vi "read_attributes.vi"(8 "error in (no error)":errorcluster, 11 "FastICA in":refnum<class "FastICA.lvclass">) -> (0 "error out":errorcluster, 2 "attributes":T1, 3 "FastICA out":refnum<class "FastICA.lvclass">)   [LabVIEW 2020, in "FastICA.lvclass"]
uses:
  FastICA.lvclass
  Controls/fast_ica_attributes.ctl
  FastICA.lvclass/FastICA.ctl
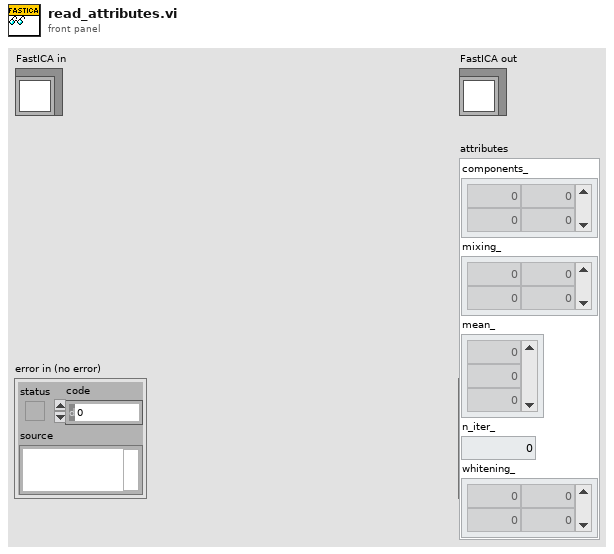
[diagram p1: front panel]
types:
  T1 = typedef "fast_ica_attributes.ctl" = cluster{"components_":dbl[][], "mixing_":dbl[][], "mean_":dbl[], "n_iter_":dbl, "whitening_":dbl[][]}
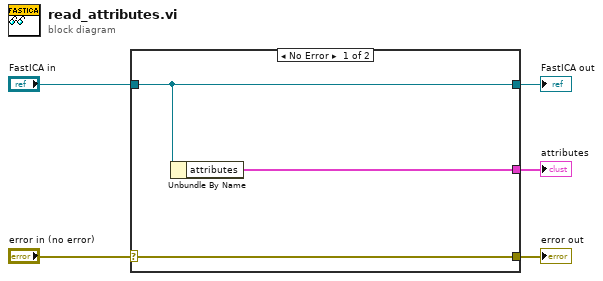
[diagram p0: block diagram]
diagram:
  n1 = case shown="No Error" "error in (no error)" {
    selector: "error in (no error)" -> [w8 w9]
    tunnel: [w8 w9] -> w4
    tunnel: [w7 w10] -> w2
    tunnel: "FastICA in" -> [w7 w10]
    tunnel: [w6 _] -> w1
    frame No Error {
      n2 = Unbundle By Name(w7) -> ("attributes"=w6:T1)
    }
    frame Error {
    }
  }
  "error out" <- w4
  "FastICA out" <- w2
  "attributes" <- w1
